vi "Parse Text then Tag.vi"(8 "Error In":errorcluster) -> (0 "Error Out":errorcluster)   [LabVIEW 2017, in "Tests.lvlib" / "Parser.lvlib"]
uses:
  Parser.lvlib
  src/Mustache/Public/Readers/Public/String/String.lvclass
  D:/Users/cfield/Code/Field R&D Services/Mustache/feature-lv-original-parser/src/Mustache/Public/Readers/Public/Abstract/Abstract.lvclass
  <vilib>/addons/_JKI Toolkits/Caraya/classes/Test/Test.lvclass
  src/Mustache/Public/Parser/Parser.lvclass
  <vilib>/addons/_JKI Toolkits/Caraya/classes/Assert/Assert.lvclass
  src/Mustache/Public/Tokens/Public/Abstract/Abstract.lvclass
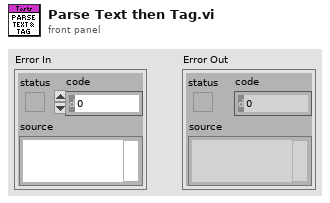
[diagram p1: front panel]
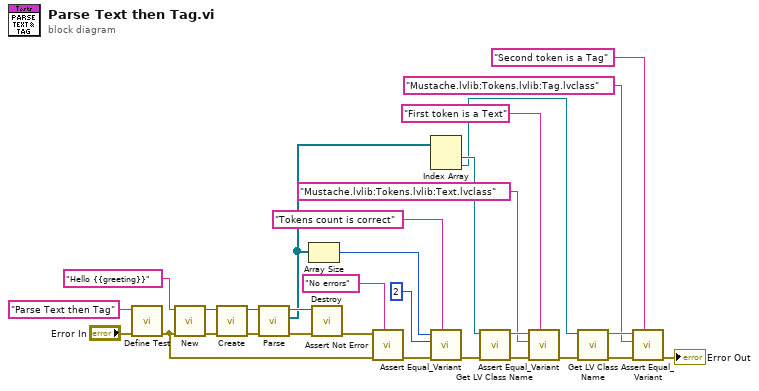
[diagram p0: block diagram]
diagram:
  n1 = call <vilib>:"Define Test.vi"("error in (no error)"="Error In", "Label (VI Title)"="Parse Text then Tag") -> ("error out"=w20:errorcluster)  [unwired: 9 in]
  n2 = call "New.vi"("Error In"=w20, "String"="Hello {{greeting}}") -> ("Error Out"=w26:errorcluster, "String"=w27:refnum<class "String.lvclass">)  [unwired: 8 in]
  n3 = call "Create.vi"("Error In"=w26, "Reader"=w27) -> ("Error Out"=w25:errorcluster, "Parser"=w24:refnum<class "Parser.lvclass">)  [unwired: 8 in]
  n4 = call "Parse.vi"("Error In"=w25, "Parser In"=w24) -> ("Error Out"=w22:errorcluster, "Tokens"=w13:refnum<class "Abstract.lvclass">[], "Parser Out"=w23:refnum<class "Parser.lvclass">)  [unwired: 7 in]
  n5 = Array Size(array=w13) -> (size(s)=w16:i32)
  n6 = call "Destroy.vi"("Error In"=w22, "Parser"=w23) -> ("Error Out"=w21:errorcluster)  [unwired: 9 in]
  n7 = call <vilib>:"Assert Not Error.vi"("Label"="No errors", "error in (no error)"=w20, "Not Error?"=w21) -> ("error out"=w18:errorcluster)  [unwired: 8 in]
  n8 = Index Array(array=w13) -> (element #1=w12:refnum<class "Abstract.lvclass">, element #2=w7:refnum<class "Abstract.lvclass">)  [unwired: 2 in]
  n9 = call <vilib>:"Assert Equal_Variant.vi"("Label"="Tokens count is correct", "error in (no error)"=w18, "Y"=2 ("size(s)"), "X"=w16) -> ("error out"=w14:errorcluster)  [unwired: 7 in]
  n10 = call <vilib>:"Get LV Class Name.vi"("error in (no error)"=w14, "object"=w12) -> ("error out"=w11:errorcluster, "class name"=w10:string)  [unwired: 8 in]
  n11 = call <vilib>:"Assert Equal_Variant.vi"("Label"="First token is a Text", "error in (no error)"=w11, "Y"="Mustache.lvlib:Tokens.lvlib:Text.lvclass", "X"=w10) -> ("error out"=w6:errorcluster)  [unwired: 7 in]
  n12 = call <vilib>:"Get LV Class Name.vi"("error in (no error)"=w6, "object"=w7) -> ("error out"=w5:errorcluster, "class name"=w4:string)  [unwired: 8 in]
  n13 = call <vilib>:"Assert Equal_Variant.vi"("Label"="Second token is a Tag", "error in (no error)"=w5, "Y"="Mustache.lvlib:Tokens.lvlib:Tag.lvclass", "X"=w4) -> ("error out"=→"Error Out":errorcluster)  [unwired: 7 in]
